vi "Enclose Selection.vi"   [LabVIEW 2019]
doc: "Demonstrates the EncloseSelection method in VI Scripting to programmatically create a structure around the selected part of the block diagram."
uses:
  <vilib>/Utility/traverseref.llb/TRef TravTarget.ctl
  <vilib>/Utility/traverseref.llb/VI Scripting - Traverse.lvlib
panel:
  # "Overview: Demonstrates the EncloseSelection method in VI Scripting to programmatically create a structure around the selected part of the block diagram.\nInstructions:\n1. Open the block diagram of Test - Selection List Target.vi.\n2. Select at least one object on the diagram.\n2. Run this VI. The item(s) you selected will be wrapped in a Sequence structure."
types:
  T1 = typedef "TRef TravTarget.ctl" = enum16{"FP", "BD", "Other"}
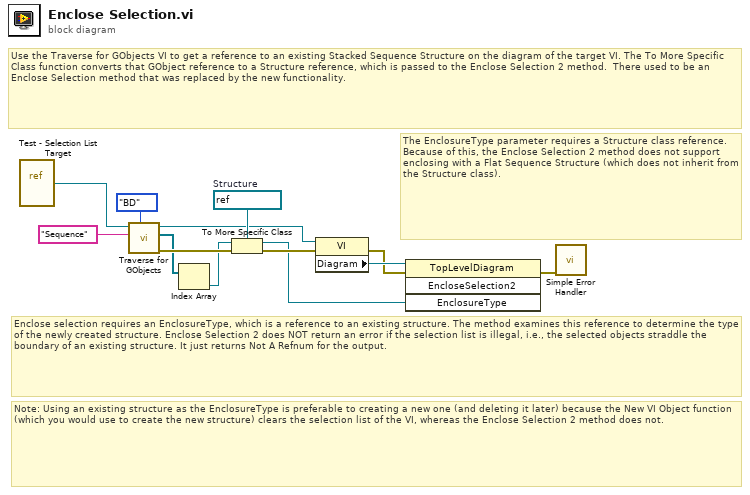
[diagram p0: block diagram]
diagram:
  w4 = refnum<vi> refnum  # Structure
  # "The EnclosureType parameter requires a Structure class reference. Because of this, the Enclose Selection 2 method does not support enclosing with a Flat Sequence Structure (which does not inherit from the Structure class)."
  # "Enclose selection requires an EnclosureType, which is a reference to an existing structure. The method examines this reference to determine the type of the newly created structure. Enclose Selection 2 does NOT return an error if the selection list is illegal, i.e., the selected objects straddle the boundary of an existing structure. It just returns Not A Refnum for the output."
  # "Use the Traverse for GObjects VI to get a reference to an existing Stacked Sequence Structure on the diagram of the target VI. The To More Specific Class function converts that GObject reference to a Structure reference, which is passed to the Enclose Selection 2 method.  There used to be an Enclose Selection method that was replaced by the new functionality."
  # "Note: Using an existing structure as the EnclosureType is preferable to creating a new one (and deleting it later) because the New VI Object function (which you would use to create the new structure) clears the selection list of the VI, whereas the Enclose Selection 2 method does not."
  n1 = vi-ref "Test - Selection List Target.vi"() -> (w10:refnum<vi>)
  n2 = call <vilib>:"Traverse for GObjects.vi"("Traverse Target"=TRef_TravTarget."BD", "Class Name"="Sequence", "VI Refnum"=w10) -> ("error out"=w11:errorcluster, "References"=w6:refnum<vi>[], "dup VI Refnum"=w3:refnum<vi>)  [unwired: 5 in, 1 out]
  n3 = Index Array(array=w6) -> (element=w5:refnum<vi>)  [unwired: 1 in]
  n4 = To More Specific Class(target class=w4, reference=w5, error in=w11) -> (specific class reference=w2:refnum<vi>, error out=w7:errorcluster)
  n5 = property class="VI"(reference=w3, error in=w7) -> (error out=w12:errorcluster, "Diagram"=w13:refnum<vi>)  [unwired: 1 out]
  n6 = invoke class="TopLevelDiagram" method="EncloseSelection2"(reference=w13, error in=w12, "EnclosureType"=w2) -> (error out=w1:errorcluster)  [unwired: 1 in, 3 out]
  n7 = call <vilib>:"Simple Error Handler.vi"("error in (no error)"=w1) -> ()  [unwired: 4 in, 5 out]
